vi "File.Rotate.Execute Rotation Task.vi"(11 "Task":T1) -> (0 "error out":errorcluster)   [LabVIEW 2018]
uses:
  <vilib>/KATE/Files/File Utils.lvlib
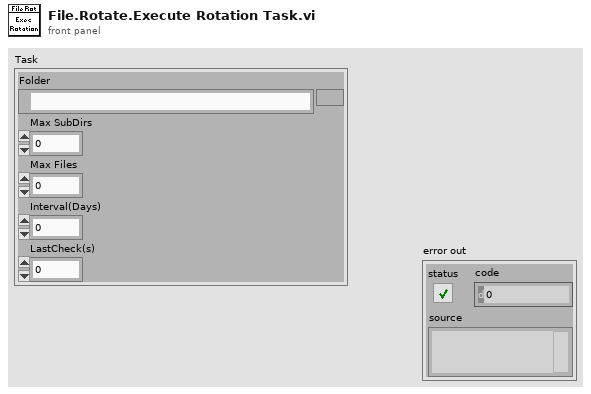
[diagram p1: front panel]
types:
  T1 = cluster{"Folder":path, "Max SubDirs":i32, "Max Files":i32, "Interval(Days)":dbl, "LastCheck(s)":dbl}
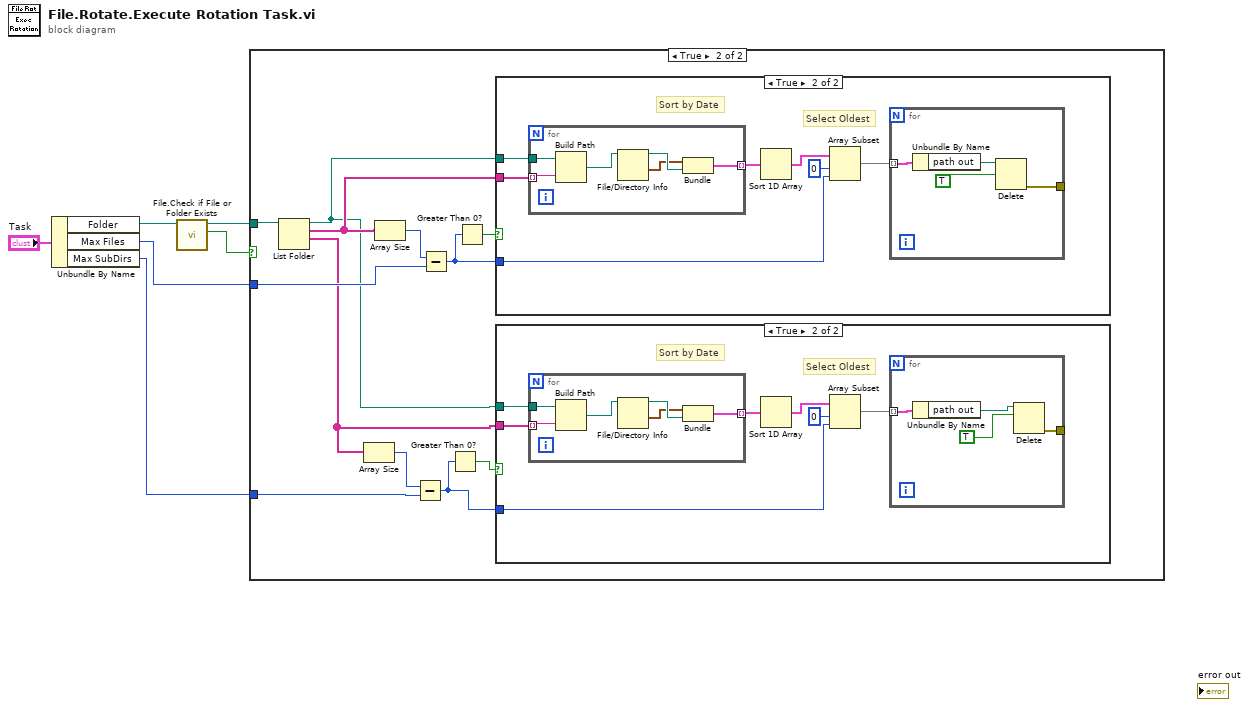
[diagram p0: block diagram]
diagram:
  n1 = Unbundle By Name("Task") -> ("Folder"=w5:path, "Max Files"=w2:i32, "Max SubDirs"=w1:i32)
  n2 = call <vilib>:"File.Check if File or Folder Exists.vi"("Path"=w5) -> ("Exists"=w3:bool, "Dup Path"=w4:path)  [unwired: 6 in, 3 out]
  n3 = case shown="True" w3 {
    tunnel: w4 -> [_ w18]
    tunnel: w2 -> [_ w11]
    tunnel: w1 -> [_ w15]
    frame False {
      # "TODO indicate warning"
    }
    frame True {
      n4 = List Folder(path=w18) -> (path out=w10:path, filenames=w17:string[], folder names=w9:string[])  [unwired: 3 in, 1 out]
      n5 = Array Size(array=w9) -> (size(s)=w16:i32)
      n6 = Array Size(array=w17) -> (size(s)=w12:i32)
      n7 = Subtract(x=w16, y=w15) -> (x-y=w7:i32)
      n8 = Subtract(x=w12, y=w11) -> (x-y=w13:i32)
      n9 = Greater Than 0?(x=w7) -> (x > 0?=w8:bool)
      n10 = Greater Than 0?(x=w13) -> (x > 0?=w14:bool)
      n11 = case shown="True" w14 {
        tunnel: w10 -> [_ w42]
        tunnel: w17 -> [_ w41]
        tunnel: w13 -> [_ w38]
        frame False {
        }
        frame True {
          # "Select Oldest"
          # "Sort by Date"
          n12 = for {
            tunnel: w42 -> [w52]
            tunnel: w41 -> [w51] mode=indexing
            tunnel: [w47] -> w40 mode=indexing
            n13 = Build Path(base path=w52, name or relative path=w51) -> (appended path=w50:path)
            n14 = File/Directory Info(path=w50) -> (path out=w49:path, last mod=w48:timestamp)  [unwired: 1 in, 5 out]
            n15 = Bundle("last mod"=w48, "path out"=w49) -> (w47:cluster{"last mod":timestamp, "path out":path})  [unwired: 1 in]
          }
          n16 = Sort 1D Array(array=w40) -> (sorted array=w39:cluster{"last mod":timestamp, "path out":path}[])
          n17 = Array Subset(array=w39, index=0, length=w38) -> (w36:cluster{"last mod":timestamp, "path out":path}[])
          n18 = for {
            tunnel: w36 -> [w46] mode=indexing
            tunnel: [w44] -> _
            n19 = Unbundle By Name(w46) -> ("path out"=w45:path)
            n20 = Delete(path (use dialog)=w45, entire hierarchy (F)=TRUE) -> (error out=w44:errorcluster)  [unwired: 3 in, 2 out]
          }
        }
      }
      n21 = case shown="True" w8 {
        tunnel: w10 -> [_ w25]
        tunnel: w9 -> [_ w24]
        tunnel: w7 -> [_ w19]
        frame False {
        }
        frame True {
          # "Select Oldest"
          # "Sort by Date"
          n22 = for {
            tunnel: w25 -> [w35]
            tunnel: w24 -> [w34] mode=indexing
            tunnel: [w30] -> w23 mode=indexing
            n23 = Build Path(base path=w35, name or relative path=w34) -> (appended path=w33:path)
            n24 = File/Directory Info(path=w33) -> (path out=w32:path, last mod=w31:timestamp)  [unwired: 1 in, 5 out]
            n25 = Bundle("last mod"=w31, "path out"=w32) -> (w30:cluster{"last mod":timestamp, "path out":path})  [unwired: 1 in]
          }
          n26 = Sort 1D Array(array=w23) -> (sorted array=w22:cluster{"last mod":timestamp, "path out":path}[])
          n27 = Array Subset(array=w22, index=0, length=w19) -> (w20:cluster{"last mod":timestamp, "path out":path}[])
          n28 = for {
            tunnel: w20 -> [w29] mode=indexing
            tunnel: [w26] -> _
            n29 = Unbundle By Name(w29) -> ("path out"=w28:path)
            n30 = Delete(path (use dialog)=w28, entire hierarchy (F)=TRUE) -> (error out=w26:errorcluster)  [unwired: 3 in, 2 out]
          }
        }
      }
    }
  }
